vi "Default Inspections.vi"(10 "Inspector Config in":T1) -> (2 "Inspector Config":T1)   [LabVIEW 2020, in "SoL Inspector.lvlib"]
uses:
  SoL Inspector.lvlib
  Inspector Config.ctl
  Inspection.ctl
  b6cbda09-5b6a-4ca9-8331-bd7473517a40.vi
  <vilib>/Comparison/Equal/Equal Functor/Equal Functor.lvclass
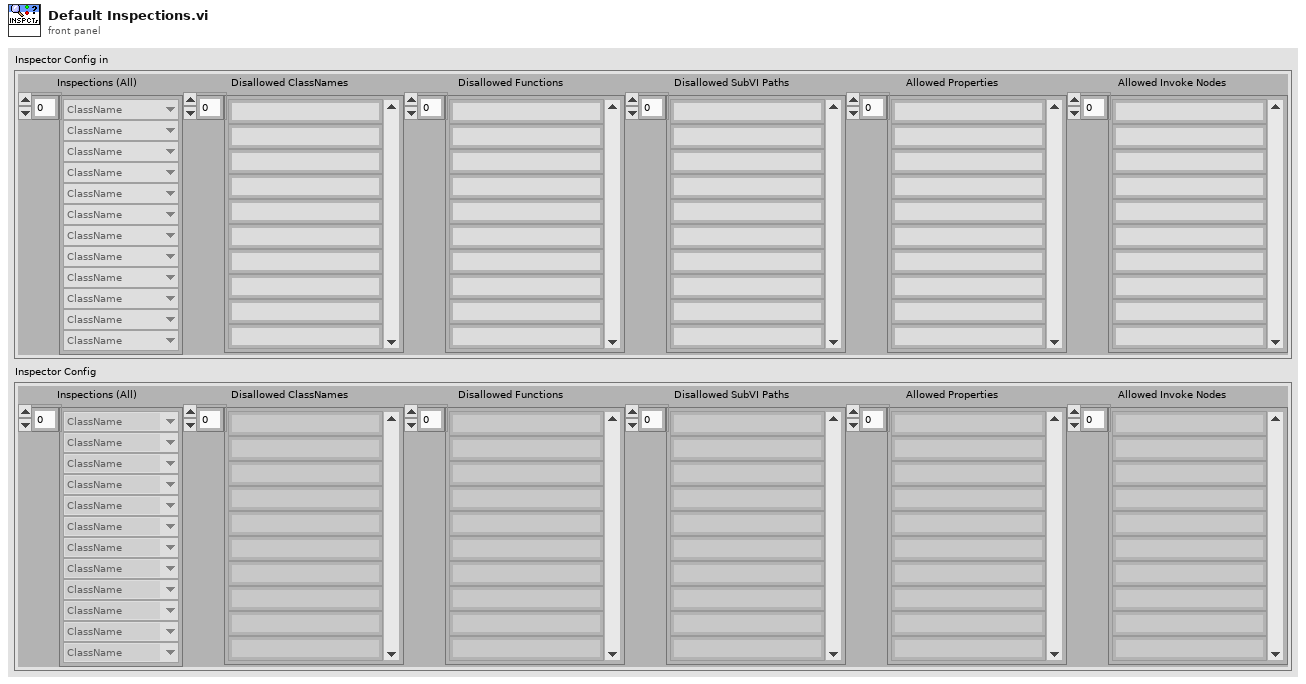
[diagram p1: front panel]
types:
  T1 = typedef "SoL Inspector.lvlib/Inspector Config.ctl" = cluster{"Inspections (All)":T2[], "Disallowed ClassNames":string[], "Disallowed Functions":string[], "Disallowed SubVI Paths":string[], "Allowed Properties":string[], "Allowed Invoke Nodes":string[]}
  T2 = typedef "SoL Inspector.lvlib/Inspection.ctl" = enum16{"ClassName", "Functions", "CallLibrary", "SubVIs", "FileIO", "Invoke Nodes", "Properties", "Growable Functions"}
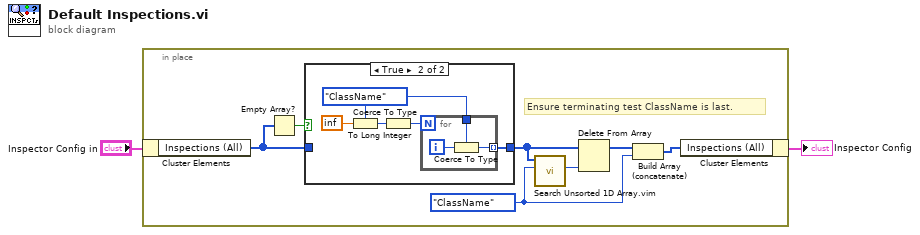
[diagram p0: block diagram]
diagram:
  n1 = in-place {
    w3 = Inspection."ClassName" ("Inspection")
    # "Ensure terminating test ClassName is last."
    n2 = in-place-cluster #1("Inspector Config in") -> ("Inspections (All)"=w8:T2[])
    n3 = Empty Array?(array=w8) -> (empty?=w9:bool)
    n4 = case shown="True" w9 {
      tunnel: w8 -> [w10 _]
      tunnel: [w10 w11] -> w7
      frame False {
      }
      frame True {
        w12 = Inspection."ClassName" ("Inspection")
        n5 = Coerce To Type(0:inf, 1:w12) -> (2:w14:T2)
        n6 = To Long Integer(number=w14) -> (32bit integer=w13:i32)
        n7 = for {
          N: w13 -> [_]
          tunnel: w12 -> [w17]
          tunnel: [w16] -> w11 mode=indexing
          i -> [w18]
          n8 = Coerce To Type(0:w18, 1:w17) -> (2:w16:T2)
        }
      }
    }
    n9 = call "Search Unsorted 1D Array.vim"("element"=w3, "unsorted 1D array"=w7) -> ("index of element"=w5:i32)  [unwired: 9 in]
    n10 = Delete From Array(array=w7, index=w5) -> (array with subset deleted=w6:T2[])  [unwired: 1 in, 1 out]
    n11 = Build Array (concatenate)(w6, w3) -> (w4:T2[])
    n12 = in-place-cluster #1("Inspections (All)"=w4) -> (→"Inspector Config":T1)
  }
